vi "filter_matrix - forvard.vi"(7 "matrix in":dbl[][](array[numeric])=array1x4097[4097 elements], 8 "forward distance":dbl, 9 "multiplication/substitution":i16(ring) items=["subst", "mult"], 10 "intensity/phase":i16(ring) items=["int", "pha"], 11 "field":T1) -> (2 "forwarded dist":dbl=1.0, 3 "field out":T1)   [LabVIEW 2012, in "Lightpipes.lvlib"]
uses:
  Lightpipes.lvlib
panel:
  out "number of columns":i32
  out "number of rows":i32
  out "matrix 1D":dbl[](array[numeric])
  out "matrix out":dbl[](array[numeric])
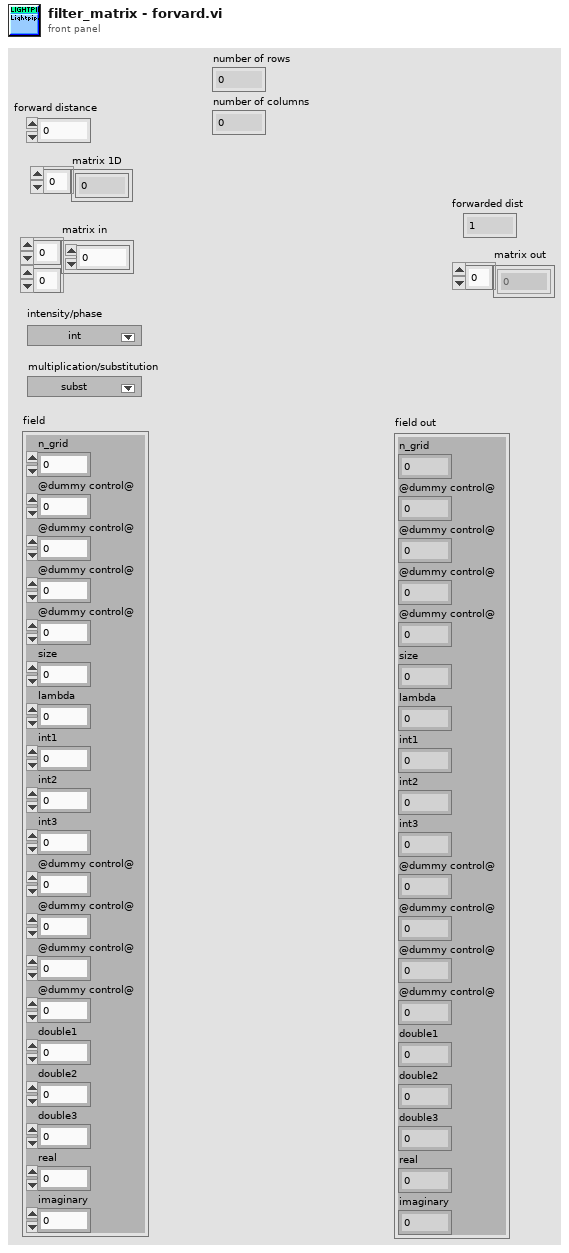
[diagram p1: front panel]
types:
  T1 = cluster{"n_grid":i32, "@dummy control@":i8, "@dummy control@":i8, "@dummy control@":i8, "@dummy control@":i8, "size":dbl, "lambda":dbl, "int1":i32, "int2":i32, "int3":i32, "@dummy control@":i8, "@dummy control@":i8, "@dummy control@":i8, "@dummy control@":i8, "double1":dbl, "double2":dbl, "double3":dbl, "real":u32, "imaginary":u32}
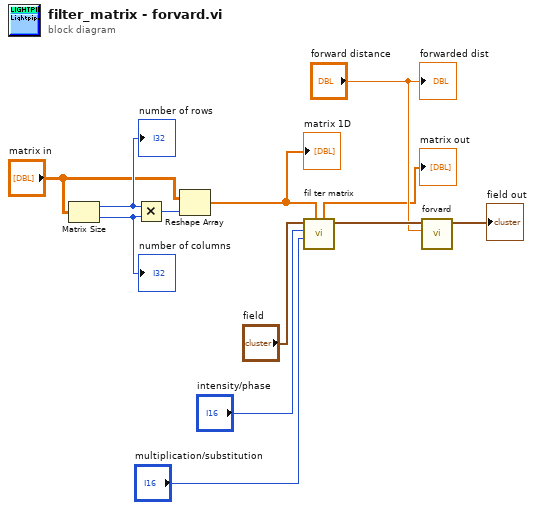
[diagram p0: block diagram]
diagram:
  n1 = Matrix Size(0:"matrix in") -> (1:w4:i32, 2:w3:i32)
  "number of rows" <- w4
  "number of columns" <- w3
  n2 = Multiply(x=w4, y=w3) -> (x*y=w1:i32)
  n3 = Reshape Array "Reshape Array"("matrix in", w1) -> (w5:dbl[])
  "matrix 1D" <- w5
  n4 = call "fil ter matrix.vi"("matrix"=w5, "multiplication/ substitution"="multiplication/substitution", "intensity / phase"="intensity/phase", "field"="field") -> ("field out"=w11:T1, "matrix out"=→"matrix out":dbl[])  [unwired: 6 in]
  n5 = call "forvard.vi"("distance"="forward distance", "field"=w11) -> ("field out"=→"field out":T1)  [unwired: 9 in]
  "forwarded dist" <- "forward distance"
